vi "No error - Tests.vi"(8 "error in (no error)":errorcluster) -> (0 "error out":errorcluster)   [LabVIEW 2017]
uses:
  System.Windows.Forms
  <vilib>/addons/_JKI Toolkits/Caraya/classes/Assert/Assert Not Error.vi
  <vilib>/addons/_JKI Toolkits/Caraya/classes/Assert/Assert Equal Value_Variant.vi
  <vilib>/addons/_JKI Toolkits/Caraya/classes/Test/Test.lvclass
  <vilib>/addons/_JKI Toolkits/Caraya/classes/Assert/Assert.lvclass
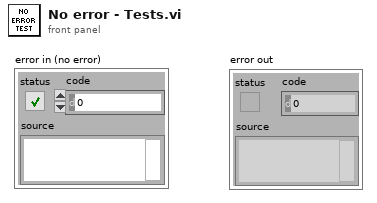
[diagram p1: front panel]
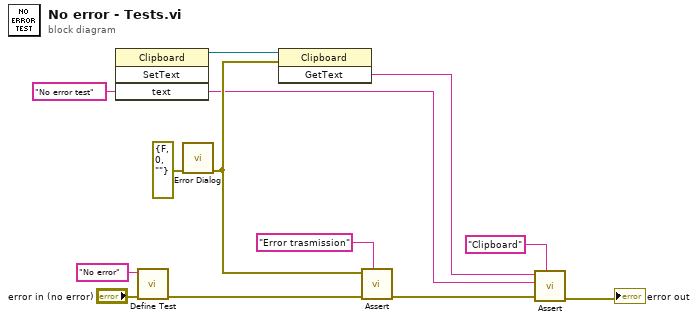
[diagram p0: block diagram]
diagram:
  w3 = "No error test" ("text")
  n1 = invoke class="Clipboard" method="SetText"("text"=w3) -> (reference out=w7:refnum<k24>)  [unwired: 3 in, 3 out]
  n2 = call <vilib>:"Define Test.vi"("error in (no error)"="error in (no error)", "Label (VI Title)"="No error") -> ("error out"=w9:errorcluster)  [unwired: 9 in]
  n3 = call "Error Dialog.vi"("error in (no error)"=errorcluster {"status"=FALSE, "code"=0, "source"=""}) -> ("error out"=w6:errorcluster)  [unwired: 10 in]
  n4 = invoke class="Clipboard" method="GetText"(reference=w7, error in=w6) -> ("GetText"=w4:string)  [unwired: 1 in, 2 out]
  n5 = call-poly <vilib>:"Assert.vi"("Label"="Error trasmission", "error in (no error)"=w9, "Not Error?"=w6) -> ("error out"=w5:errorcluster)  [unwired: 8 in]
  n6 = call-poly <vilib>:"Assert.vi"("Label"="Clipboard", "error in (no error)"=w5, "Y"=w3, "X"=w4) -> ("error out"=→"error out":errorcluster)  [unwired: 7 in]
